vi "MainWiFi.vi"() -> ()   [LabVIEW 2018]
doc: "This example sets the RS-485 transceiver control modes for the specified port and performs a serial port read, a serial port write, or a combination of these actions. If all are selected, the VI will write the data first, read data and then close the VISA session that is opened to the port. This VI will wait until the specified number of bytes is received at the port or until a termination character is received. This example will work only with National Instruments RS-485 interfaces.\n\nThis example demonstrates the transceiver control modes available when using a National Instruments RS-485 product. When connecting one or several devices via RS-485, a user may want to cut down on the amount of wiring. Alternatively, some devices offer a certain wiring configuration that you may need to match. Determine the wiring needs of the connected serial device to determine which NI RS-485 transceiver control mode to choose.\n\nWhen you are communicating with a two-wire device, National Instruments recommends that you use the two-wire Auto Control mode. This mode handles the transmitter/receiver enabling for a two-wire connection in your hardware, so it reduces the software overhead required to perform this operation in your application program."
uses:
  estados.ctl
  mensagemFila.ctl
panel:
  in  "Port":u16=555 caption="Numeric"
  in  "IP Address":string="192.168.4.1" caption="String"
  out "elements":T1[](array[typedef])
  out "# elements in queue":i32
  out "?":T2
  in  "Power":bool
  out "SP = VP\nEscravo 2":bool
  out "SP = VP\nEscravo 1":bool
  out "Waveform Chart":T3(graph)
  in  "Sensor Escravo 2":u16(ring) caption="Ring" items=["LM35", "4 - 20 mA"]
  in  "Sensor Escravo 1":u16(ring) caption="Ring" items=["LM35", "4 - 20 mA"]
  in  "Verifica Sensor sl2":bool caption="Verifica Sensor\nEscravo 2"
  in  "Verifica Sensor sl1":bool caption="Verifica Sensor\nEscravo 1"
  in  "Envia Sensor sl2":bool caption="Seta Sensor\nEscravo 2"
  in  "Envia Sensor sl1":bool caption="Seta Sensor\nEscravo 1"
  out "Status":string caption="String"
  in  "Verifica SP sl2":bool caption="Verifica SP\nEscravo 2"
  in  "Verifica SP sl1":bool caption="Verifica SP\nEscravo 1"
  in  "SP escravo 2":u16 caption="SP Escravo 2"
  in  "Envia SP sl2":bool caption="Seta SP\nEscravo 2"
  in  "Envia SP sl1":bool caption="Seta SP\nEscravo 1"
  in  "SP escravo 1":u16 caption="SP Escravo 1"
  in  "stop":bool
  in  "dado":u16=4
  in  "opcode":u8=4 format="%.0b"
  in  "addr":u8=4 format="%.0x"
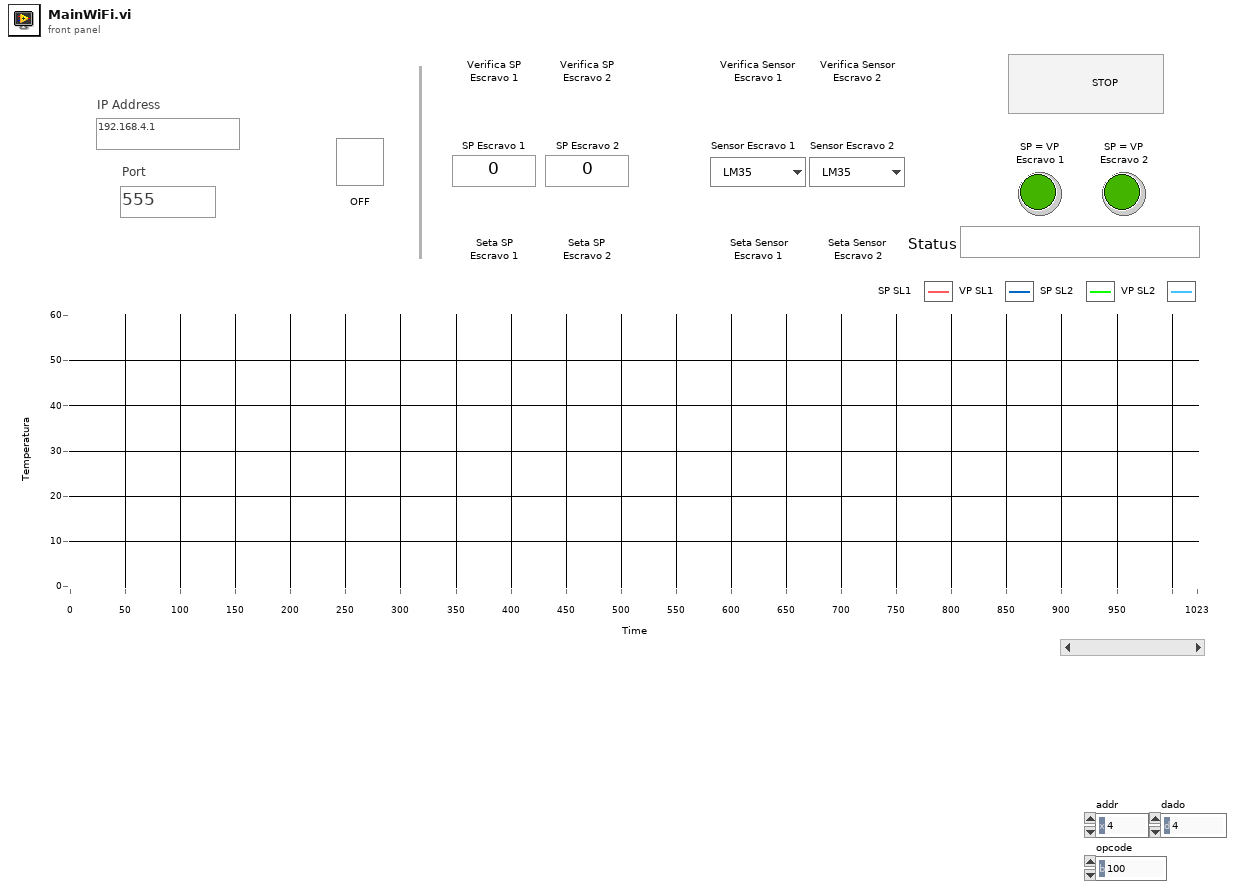
[diagram p1: front panel]
types:
  T1 = typedef "mensagemFila.ctl" = cluster{"Estado":T2, "Próximo Estado":T2, "Comando":string}
  T2 = typedef "estados.ctl" = enum16{"Idle", "Inicializa conexão", "Monta comando", "Envia comando", "Recebe resposta 1 escravo", "Recebe resposta 2 escravos", "Trata respostas", "Trata respostas 2 Escravos", "Encerra conexão", "Erro", "Stop", "Atualiza UI"}
  T3 = cluster{"plot 0":dbl, "plot 1":dbl, "plot 2":dbl, "plot 3":dbl}
  T4 = cluster{"SP escravo 1":refnum<vi>, "SP escravo 2":refnum<vi>, "Sensor Escravo 1":refnum<vi>, "Sensor Escravo 2":refnum<vi>, "SP = VP\nEscravo 1":refnum<vi>, "SP = VP\nEscravo 2":refnum<vi>, "Waveform Chart":refnum<vi>}
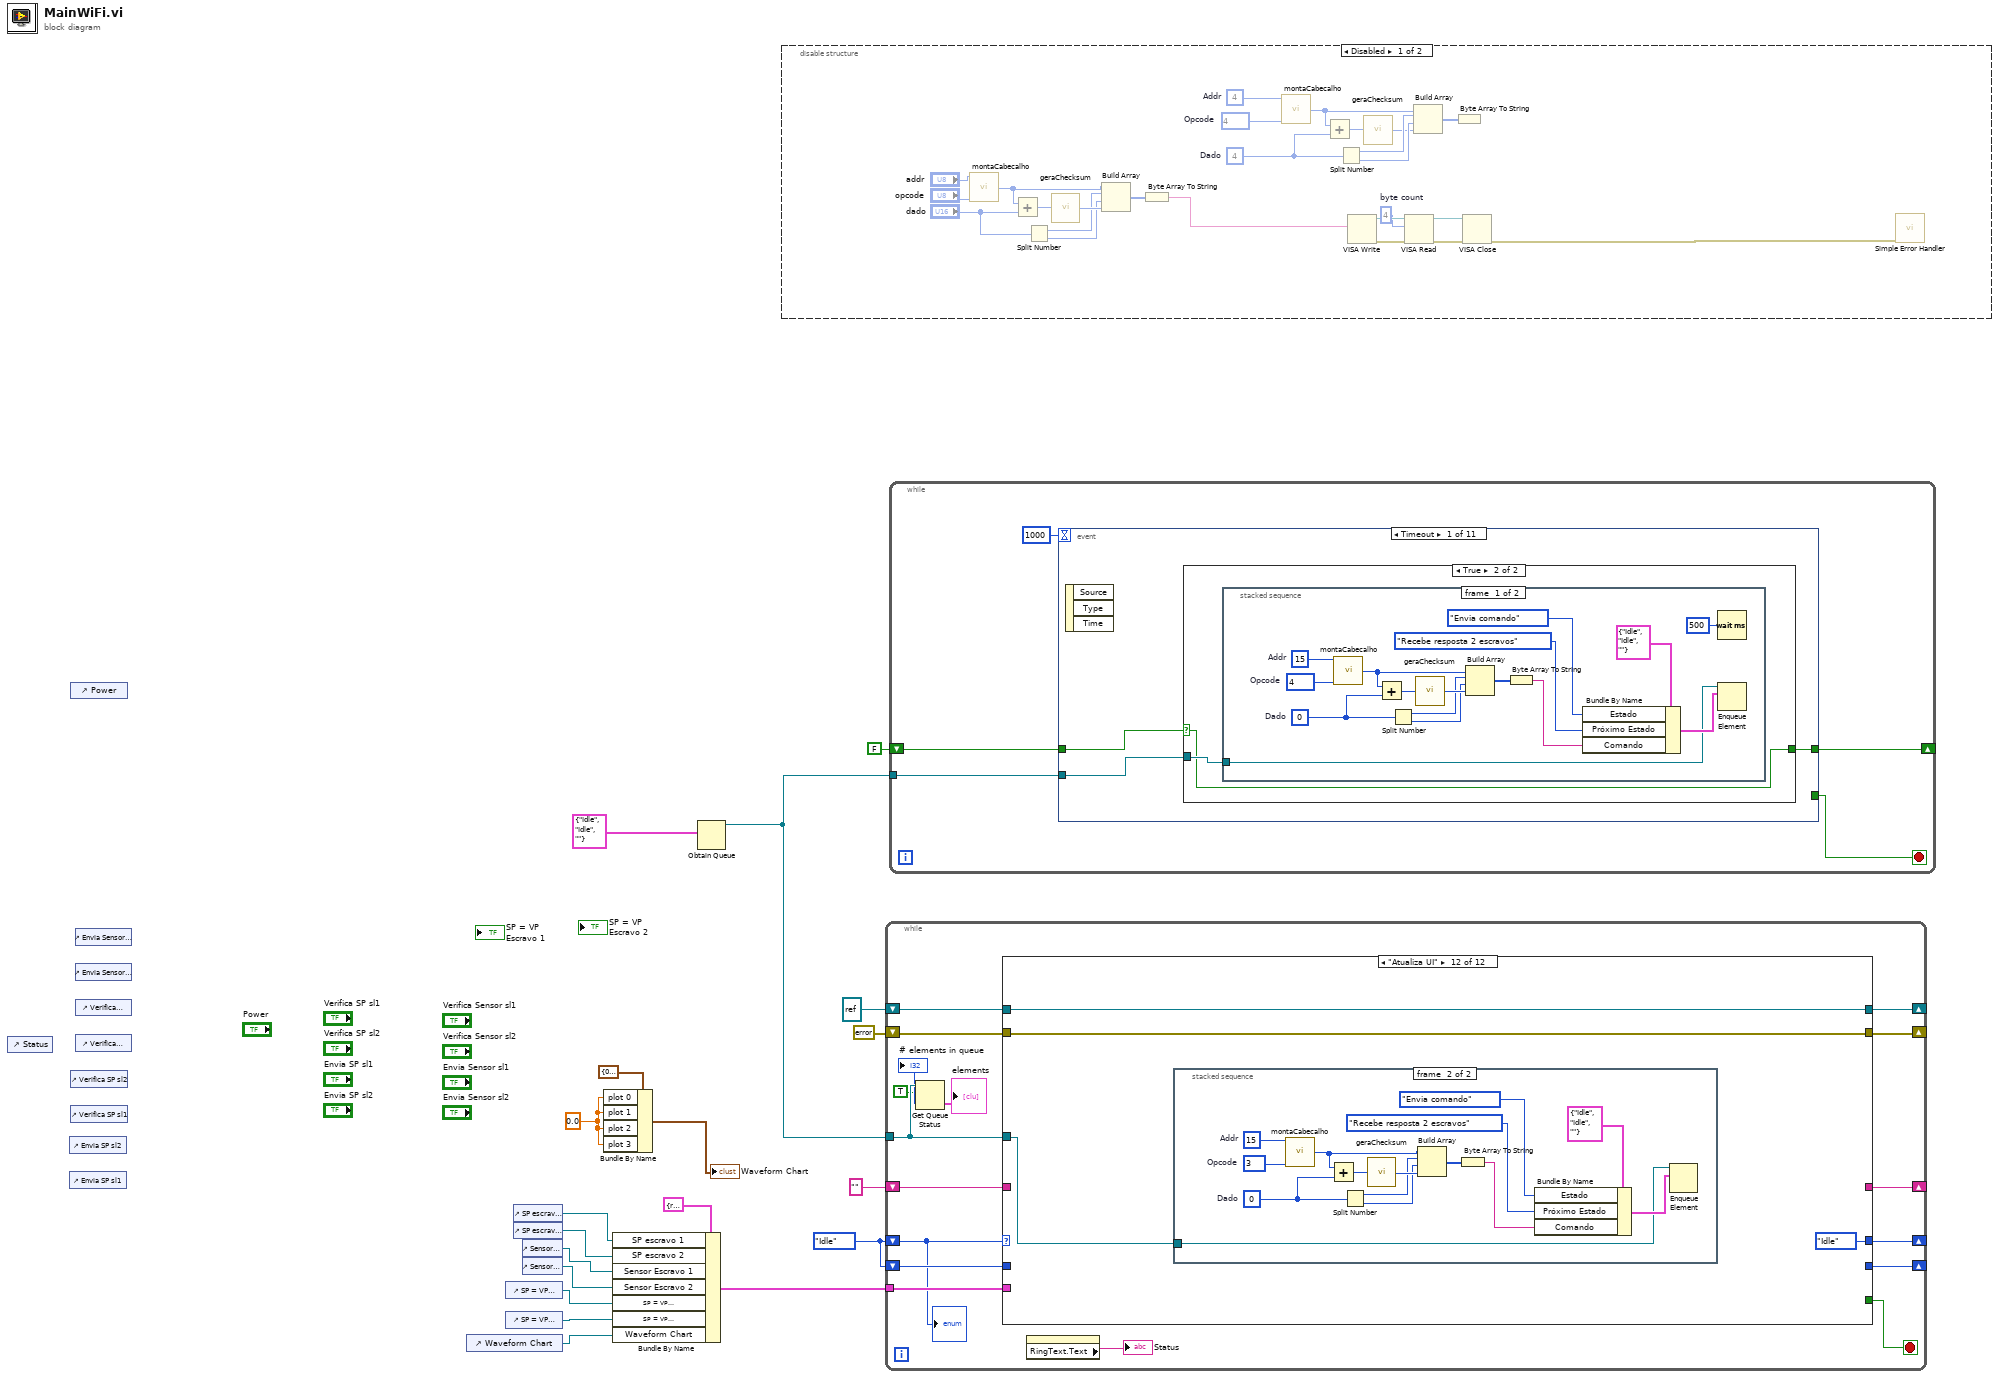
[diagram p0: block diagram]
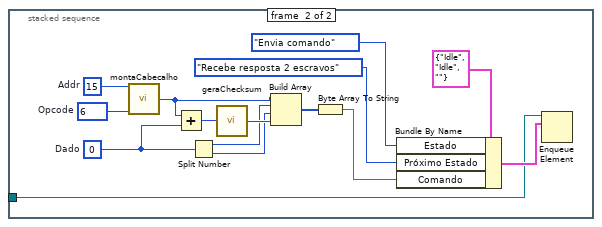
[diagram p4: hidden frame]
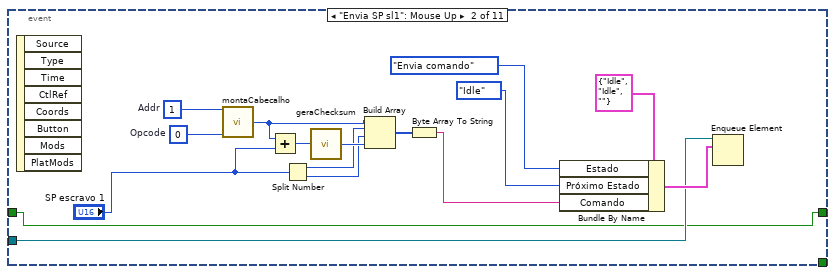
[diagram p5: hidden frame]
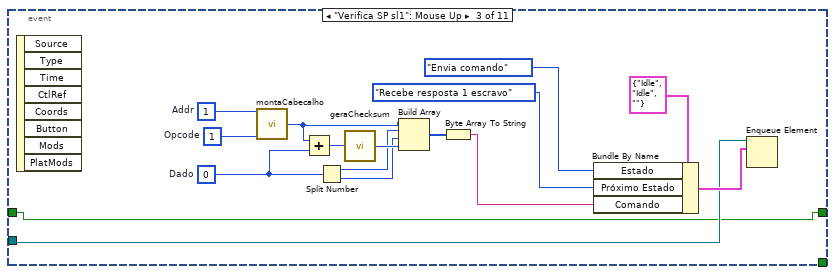
[diagram p6: hidden frame]
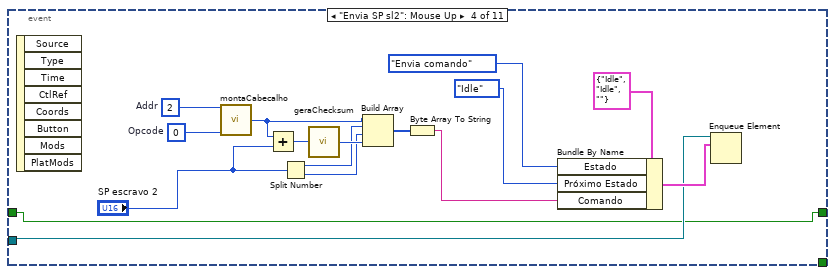
[diagram p7: hidden frame]
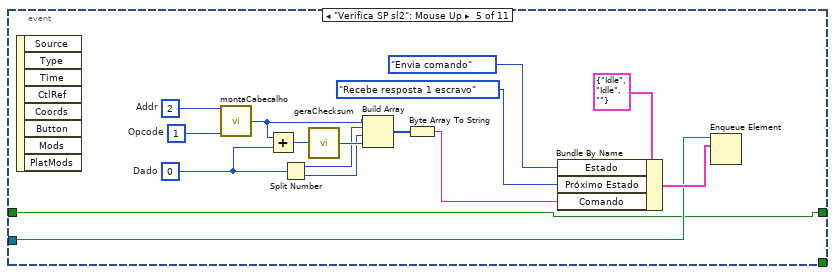
[diagram p8: hidden frame]
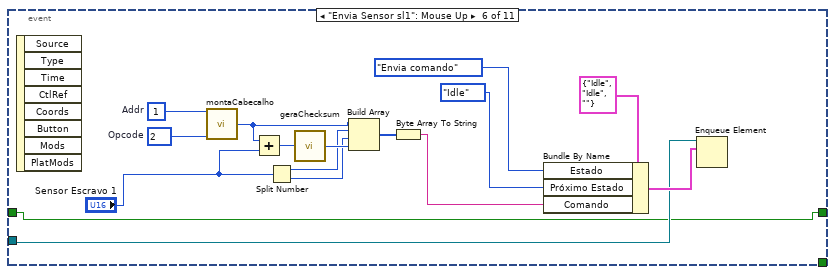
[diagram p9: hidden frame]
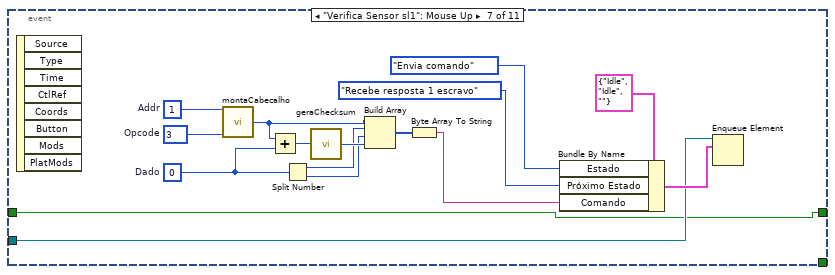
[diagram p10: hidden frame]
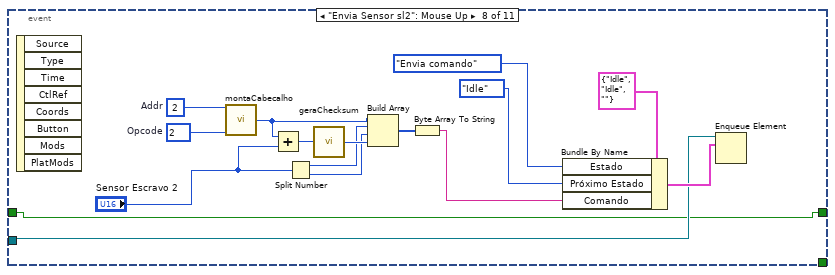
[diagram p11: hidden frame]
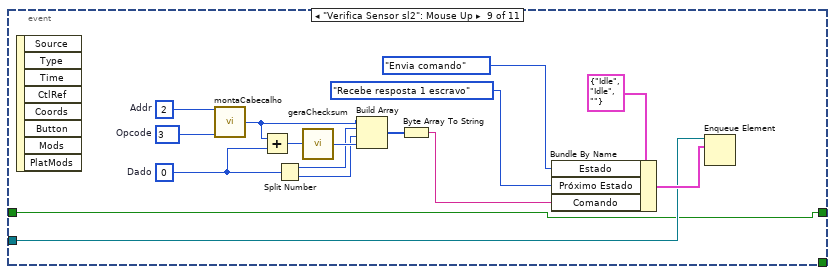
[diagram p12: hidden frame]
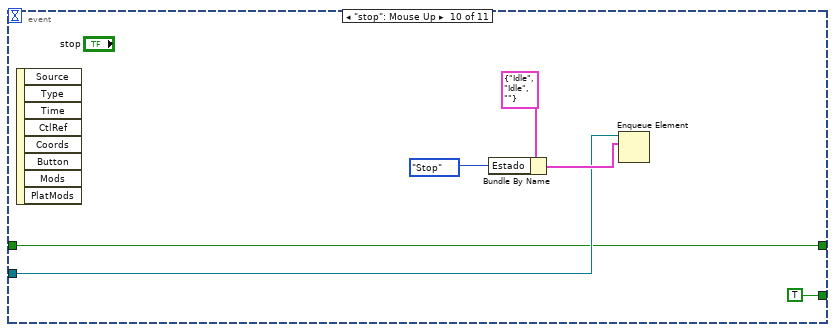
[diagram p13: hidden frame]
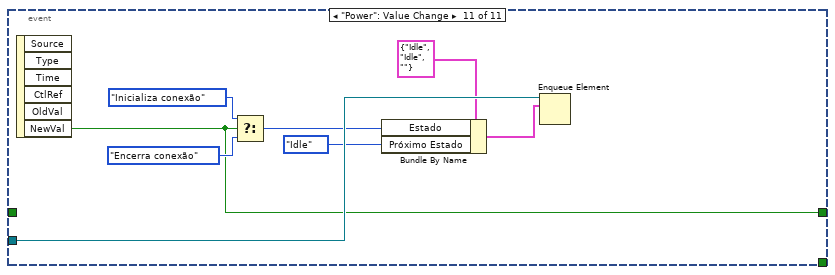
[diagram p14: hidden frame]
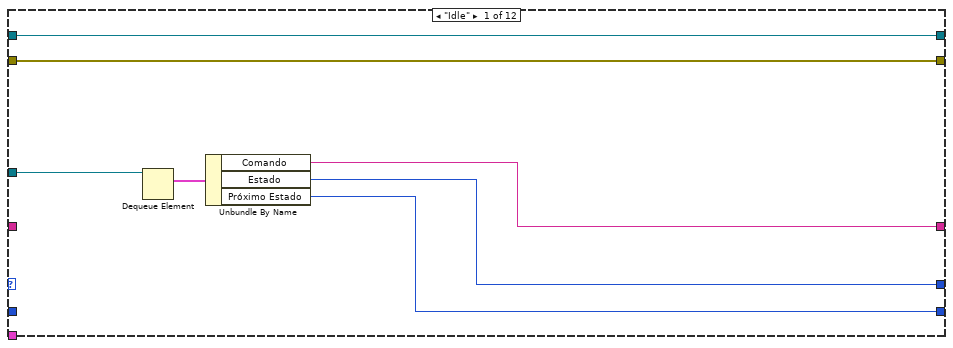
[diagram p15: hidden frame]
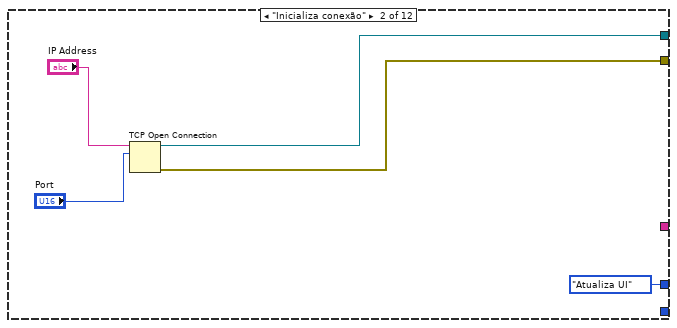
[diagram p16: hidden frame]
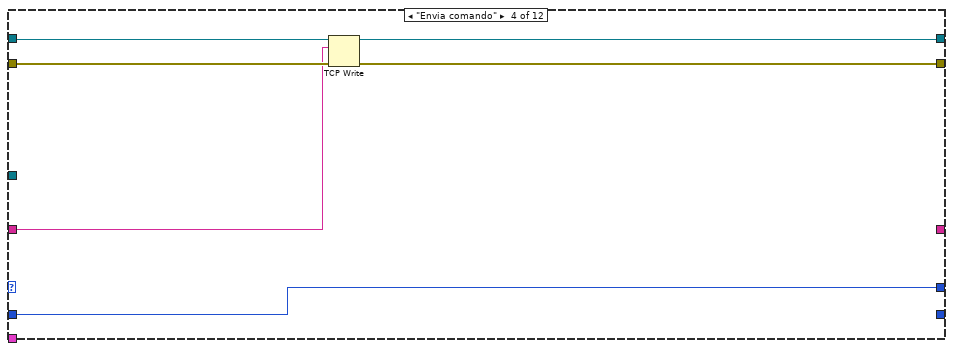
[diagram p18: hidden frame]
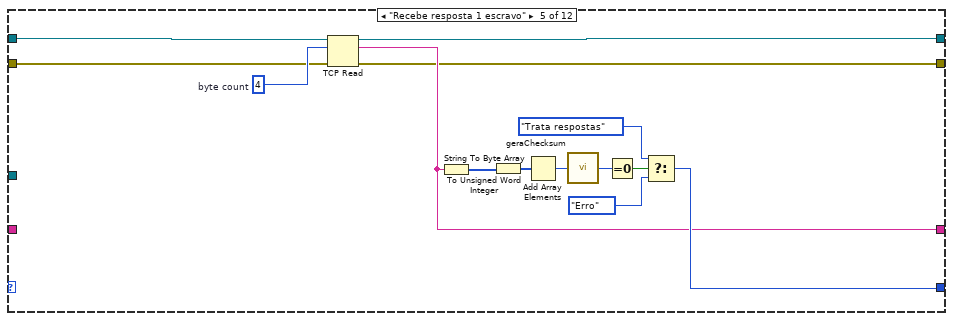
[diagram p19: hidden frame]
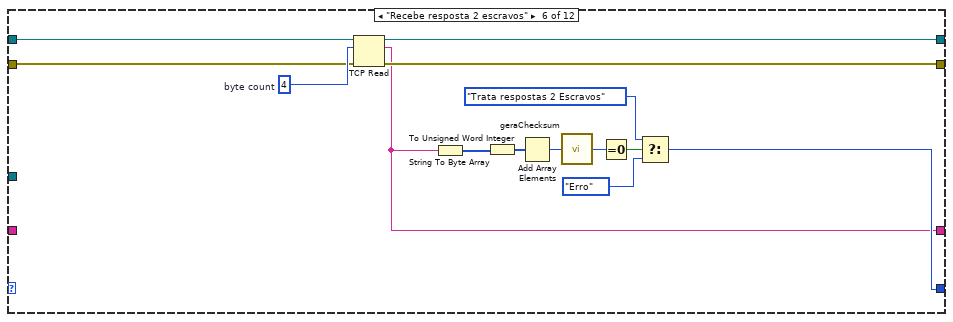
[diagram p20: hidden frame]
diagram:
  w3 = 0.0 ("element")
  w2 = estados."Idle"
  n1 = control-ref of="Status"() -> ()  [unwired: 1 out]
  n2 = control-ref of="Envia SP sl2"() -> ()  [unwired: 1 out]
  n3 = control-ref of="Envia SP sl1"() -> ()  [unwired: 1 out]
  n4 = control-ref of="Power"() -> ()  [unwired: 1 out]
  n5 = control-ref of="Verifica SP sl2"() -> ()  [unwired: 1 out]
  n6 = control-ref of="Verifica SP sl1"() -> ()  [unwired: 1 out]
  n7 = control-ref of="Envia Sensor sl2"() -> ()  [unwired: 1 out]
  n8 = control-ref of="Envia Sensor sl1"() -> ()  [unwired: 1 out]
  n9 = control-ref of="Verifica Sensor sl2"() -> ()  [unwired: 1 out]
  n10 = control-ref of="Verifica Sensor sl1"() -> ()  [unwired: 1 out]
  n11 = control-ref of="Waveform Chart"() -> (w7:refnum<vi>)
  n12 = control-ref of="SP = VP\nEscravo 1"() -> (w9:refnum<vi>)
  n13 = control-ref of="SP = VP\nEscravo 2"() -> (w8:refnum<vi>)
  n14 = control-ref of="SP escravo 1"() -> (w13:refnum<vi>)
  n15 = control-ref of="SP escravo 2"() -> (w12:refnum<vi>)
  n16 = control-ref of="Sensor Escravo 1"() -> (w11:refnum<vi>)
  n17 = control-ref of="Sensor Escravo 2"() -> (w10:refnum<vi>)
  n18 = Bundle By Name(cluster=T3 {"plot 0"=0.0, "plot 1"=0.0, "plot 2"=0.0, "plot 3"=0.0} ("input cluster"), "plot 0"=w3, "plot 1"=w3, "plot 2"=w3, "plot 3"=w3) -> (→"Waveform Chart":T3)
  n19 = Bundle By Name(cluster=T4 {"SP escravo 1"=refnum, "SP escravo 2"=refnum, "Sensor Escravo 1"=refnum, "Sensor Escravo 2"=refnum, "SP = VP\nEscravo 1"=refnum, "SP = VP\nEscravo 2"=refnum, "Waveform Chart"=refnum}, "SP escravo 1"=w13, "SP escravo 2"=w12, "Sensor Escravo 1"=w11, "Sensor Escravo 2"=w10, "SP = VP\nEscravo 1"=w9, "SP = VP\nEscravo 2"=w8, "Waveform Chart"=w7) -> (w6:T4)
  n20 = Obtain Queue(element data type=T1 {"Estado"=enum."Idle", "Próximo Estado"=enum."Idle", "Comando"=""}) -> (queue out=w17:refnum<queue>)  [unwired: 4 in, 2 out]
  n21 = disable-structure shown="Disabled" {
    frame Disabled {
      w26 = u8 4  # Addr
      w27 = u8 4  # Opcode
      w23 = u16 4  # Dado
      w39 = u32 4  # byte count
      n22 = call "montaCabecalho.vi"("addr"="addr", "opcode"="opcode") -> ("Cabeçalho"=w30:u8)  [unwired: 13 in]
      n23 = Add(x=w30, y="dado") -> (x+y=w36:u16)
      n24 = Split Number(x="dado") -> (hi(x)=w34:u8, lo(x)=w33:u8)
      n25 = call "geraChecksum.vi"("Soma"=w36) -> ("checksum"=w38:u8)  [unwired: 14 in]
      n26 = Build Array(w30, w34, w33, w38) -> (w37:u8[])
      n27 = Byte Array To String(unsigned byte array=w37) -> (string=w29:string)
      n28 = call "montaCabecalho.vi"("addr"=w26, "opcode"=w27) -> ("Cabeçalho"=w28:u8)  [unwired: 13 in]
      n29 = Add(x=w28, y=w23) -> (x+y=w22:u16)
      n30 = Split Number(x=w23) -> (hi(x)=w24:u8, lo(x)=w25:u8)
      n31 = VISA Write(write buffer=w29) -> (VISA resource name out=w44:refnum<visa-resource-name>, error out=w41:errorcluster)  [unwired: 2 in, 1 out]
      n32 = call "geraChecksum.vi"("Soma"=w22) -> ("checksum"=w20:u8)  [unwired: 14 in]
      n33 = VISA Read(VISA resource name=w44, byte count=w39, error in (no error)=w41) -> (VISA resource name out=w42:refnum<visa-resource-name>, error out=w43:errorcluster)  [unwired: 2 out]
      n34 = Build Array(w28, w24, w25, w20) -> (w21:u8[])
      n35 = Byte Array To String(unsigned byte array=w21) -> ()  [unwired: 1 out]
      n36 = VISA Close(VISA resource name=w42, error in (no error)=w43) -> (error out=w40:errorcluster)
      n37 = call <vilib>:"Simple Error Handler.vi"("error in (no error)"=w40) -> ()  [unwired: 1 in, 8 out]
    }
    frame Enabled {
    }
  }
  n38 = while {
    shift-right: [w59] -> _
    shift-left: w2 -> [w50]
    shift-right: [w58] -> _
    shift-left: errorcluster {"status"=FALSE, "code"=0, "source"=""} ("error out") -> [w60]
    shift-right: [w57] -> _
    shift-left: refnum<k5> refnum ("connection ID") -> [w61]
    shift-right: [w54] -> _
    shift-left: "" ("Dado") -> [w56]
    tunnel: w17 -> [w48]
    shift-right: [w52] -> _
    shift-left: w2 -> [w53]
    tunnel: w6 -> [w51]
    stop <- w55 stop-if-true
    n39 = Get Queue Status(queue=w48, return elements? (F)=TRUE) -> (# elements in queue=→"# elements in queue":i32, elements=→"elements":T1[])  [unwired: 1 in, 6 out]
    n40 = case shown="\"Atualiza UI\"" w50 {
      tunnel: w61 -> [w67 _ w75 w81 w85 w109 w115 w132 w136 w138 w141 w148]
      tunnel: w60 -> [w68 _ w76 w82 w95 w108 w116 w133 w137 w139 w142 w147]
      tunnel: [w63 estados."Atualiza UI" _ w77 w87 w100 estados."Idle" estados."Recebe resposta 1 escravo" _ estados."Idle" _ estados."Idle"] -> w59
      tunnel: [w68 w72 w76 w79 w83 w107 w116 w133 w135 w139 w142 w147] -> w58
      tunnel: [w67 w73 w75 w80 w84 w106 w115 w132 _ w138 w141 w148] -> w57
      tunnel: w56 -> [_ _ w74 w78 _ _ w118 w124 _ _ _ _]
      tunnel: [_ _ _ _ _ _ _ _ _ _ TRUE _] -> w55
      tunnel: w48 -> [w66 _ _ _ _ _ _ _ _ _ w143 w146]
      tunnel: [w64 _ w74 _ w86 w97 _ _ _ _ _ _] -> w54
      tunnel: w53 -> [_ _ _ w77 _ _ _ _ _ _ _ _]
      tunnel: [w62 _ _ _ _ _ _ _ _ _ _ _] -> w52
      tunnel: w51 -> [_ _ _ _ _ _ w111 w123 _ _ _ _]
      frame "Idle" {
        n41 = Dequeue Element(queue=w66) -> (element=w65:T1)  [unwired: 2 in, 3 out]
        n42 = Unbundle By Name(w65) -> ("Comando"=w64:string, "Estado"=w63:T2, "Próximo Estado"=w62:T2)
      }
      frame "Inicializa conexão" {
        n43 = TCP Open Connection(address="IP Address", remote port or service name="Port") -> (connection ID=w73:refnum<k5>, error out=w72:errorcluster)  [unwired: 3 in]
      }
      frame "Monta comando" {
      }
      frame "Envia comando" {
        n44 = TCP Write(connection ID=w81, data in=w78, error in (no error)=w82) -> (connection ID out=w80:refnum<k5>, error out=w79:errorcluster)  [unwired: 1 in, 1 out]
      }
      frame "Recebe resposta 1 escravo" {
        w96 = u32 4  # byte count
        n45 = TCP Read(connection ID=w85, bytes to read=w96, error in (no error)=w95) -> (connection ID out=w84:refnum<k5>, data out=w86:string, error out=w83:errorcluster)  [unwired: 2 in]
        n46 = String To Byte Array(string=w86) -> (unsigned byte array=w93:u8[])
        n47 = To Unsigned Word Integer(number=w93) -> (unsigned 16bit integer=w94:u16[])
        n48 = Add Array Elements(numeric array=w94) -> (sum=w92:u16)
        n49 = call "geraChecksum.vi"("Soma"=w92) -> ("checksum"=w91:u8)  [unwired: 14 in]
        n50 = Equal To 0?(x=w91) -> (x = 0?=w90:bool)
        n51 = Select(t=estados."Trata respostas", s=w90, f=estados."Erro") -> (s? t:f=w87:T2)
      }
      frame "Recebe resposta 2 escravos" {
        w110 = u32 4  # byte count
        n52 = TCP Read(connection ID=w109, bytes to read=w110, error in (no error)=w108) -> (connection ID out=w106:refnum<k5>, data out=w97:string, error out=w107:errorcluster)  [unwired: 2 in]
        n53 = String To Byte Array(string=w97) -> (unsigned byte array=w104:u8[])
        n54 = To Unsigned Word Integer(number=w104) -> (unsigned 16bit integer=w105:u16[])
        n55 = Add Array Elements(numeric array=w105) -> (sum=w103:u16)
        n56 = call "geraChecksum.vi"("Soma"=w103) -> ("checksum"=w102:u8)  [unwired: 14 in]
        n57 = Equal To 0?(x=w102) -> (x = 0?=w101:bool)
        n58 = Select(t=estados."Trata respostas 2 Escravos", s=w101, f=estados."Erro") -> (s? t:f=w100:T2)
      }
      frame "Trata respostas" {
        n59 = String To Byte Array(string=w118) -> (unsigned byte array=w122:u8[])
        n60 = Index Array(array=w122) -> (element #1=w121:u8, element #2=w120:u8, element #3=w119:u8)  [unwired: 3 in]
        n61 = call "desmontaCabecalho.vi"("cabeçalho"=w121) -> ("addr"=w112:u8, "opcode"=w113:u8)  [unwired: 13 in]
        n62 = Join Numbers(hi=w120, lo=w119) -> ((hi.lo)=w114:u16)
        n63 = call "trataMsg.vi"("addr"=w112, "opcode"=w113, "dado"=w114, "ClusterUI"=w111) -> ()  [unwired: 12 in]
      }
      frame "Trata respostas 2 Escravos" {
        n64 = String To Byte Array(string=w124) -> (unsigned byte array=w131:u8[])
        n65 = Index Array(array=w131) -> (element #1=w130:u8, element #2=w129:u8, element #3=w128:u8)  [unwired: 3 in]
        n66 = call "desmontaCabecalho.vi"("cabeçalho"=w130) -> ("addr"=w125:u8, "opcode"=w126:u8)  [unwired: 13 in]
        n67 = Join Numbers(hi=w129, lo=w128) -> ((hi.lo)=w127:u16)
        n68 = call "trataMsg.vi"("addr"=w125, "opcode"=w126, "dado"=w127, "ClusterUI"=w123) -> ()  [unwired: 12 in]
      }
      frame "Encerra conexão" {
        n69 = TCP Close Connection(connection ID=w136, error in (no error)=w137) -> (error out=w135:errorcluster)  [unwired: 1 in, 1 out]
      }
      frame "Erro" {
      }
      frame "Stop" {
        n70 = Release Queue(queue=w143) -> ()  [unwired: 2 in, 3 out]
      }
      frame "Atualiza UI" {
        n71 = stacked-sequence {
          tunnel: w146 -> [w163 w178]
          frame #0 {
            w155 = u8 15  # Addr
            w154 = u8 1  # Opcode
            w158 = u16 0  # Dado
            n72 = call "montaCabecalho.vi"("addr"=w155, "opcode"=w154) -> ("Cabeçalho"=w153:u8)  [unwired: 13 in]
            n73 = Add(x=w153, y=w158) -> (x+y=w159:u16)
            n74 = Split Number(x=w158) -> (hi(x)=w157:u8, lo(x)=w156:u8)
            n75 = call "geraChecksum.vi"("Soma"=w159) -> ("checksum"=w161:u8)  [unwired: 14 in]
            n76 = Build Array(w153, w157, w156, w161) -> (w160:u8[])
            n77 = Byte Array To String(unsigned byte array=w160) -> (string=w151:string)
            n78 = Bundle By Name(cluster=T1 {"Estado"=enum."Idle", "Próximo Estado"=enum."Idle", "Comando"=""}, "Estado"=estados."Envia comando", "Próximo Estado"=estados."Recebe resposta 2 escravos" ("Estado"), "Comando"=w151) -> (w164:T1)
            n79 = Wait (ms)(milliseconds to wait=u32 500) -> ()  [unwired: 1 out]
            n80 = Enqueue Element(queue=w163, element=w164) -> ()  [unwired: 2 in, 3 out]
          }
          frame #1 {
            w170 = u8 15  # Addr
            w169 = u8 3  # Opcode
            w173 = u16 0  # Dado
            n81 = call "montaCabecalho.vi"("addr"=w170, "opcode"=w169) -> ("Cabeçalho"=w168:u8)  [unwired: 13 in]
            n82 = Add(x=w168, y=w173) -> (x+y=w174:u16)
            n83 = Split Number(x=w173) -> (hi(x)=w172:u8, lo(x)=w171:u8)
            n84 = call "geraChecksum.vi"("Soma"=w174) -> ("checksum"=w176:u8)  [unwired: 14 in]
            n85 = Build Array(w168, w172, w171, w176) -> (w175:u8[])
            n86 = Byte Array To String(unsigned byte array=w175) -> (string=w166:string)
            n87 = Bundle By Name(cluster=T1 {"Estado"=enum."Idle", "Próximo Estado"=enum."Idle", "Comando"=""}, "Estado"=estados."Envia comando", "Próximo Estado"=estados."Recebe resposta 2 escravos" ("Estado"), "Comando"=w166) -> (w179:T1)
            n88 = Enqueue Element(queue=w178, element=w179) -> ()  [unwired: 2 in, 3 out]
          }
        }
      }
    }
    n89 = property class="Enum (strict)"() -> ("RingText.Text"=→"Status":string)  [unwired: 2 in, 2 out]
    "?" <- w50
  }
  n90 = while {
    tunnel: w17 -> [w183]
    shift-right: [w181] -> _
    shift-left: FALSE ("NewVal") -> [w180]
    stop <- w184 stop-if-true
    n91 = event shown="[0] Timeout" {
      selector: _ -> [_ _ _ _ _ _ _ _ _ _ _]
      dyn-events: _ -> [_ _ _ _ _ _ _ _ _ _ _]
      timeout: 1000 -> [_ _ _ _ _ _ _ _ _ _ _]
      tunnel: [_ _ _ _ _ _ _ _ _ TRUE _] -> w184
      tunnel: w183 -> [w187 w224 w239 w256 w271 w288 w303 w320 w335 w351 w361]
      tunnel: [w185 w222 w238 w254 w270 w286 w302 w318 w334 w350 w356] -> w181
      tunnel: w180 -> [w186 w222 w238 w254 w270 w286 w302 w318 w334 w350 _]
      event Timeout {
        n92 = event-data() -> ()  [unwired: 1 in, 3 out]
        n93 = case shown="True" w186 {
          selector: w186 -> [w188 w189]
          tunnel: w187 -> [_ w190]
          tunnel: [w188 w189] -> w185
          frame False {
          }
          frame True {
            n94 = stacked-sequence {
              tunnel: w190 -> [w205 w220]
              frame #0 {
                w197 = u8 15  # Addr
                w196 = u8 4  # Opcode
                w200 = u16 0  # Dado
                n95 = call "montaCabecalho.vi"("addr"=w197, "opcode"=w196) -> ("Cabeçalho"=w195:u8)  [unwired: 13 in]
                n96 = Add(x=w195, y=w200) -> (x+y=w201:u16)
                n97 = Split Number(x=w200) -> (hi(x)=w199:u8, lo(x)=w198:u8)
                n98 = call "geraChecksum.vi"("Soma"=w201) -> ("checksum"=w203:u8)  [unwired: 14 in]
                n99 = Build Array(w195, w199, w198, w203) -> (w202:u8[])
                n100 = Byte Array To String(unsigned byte array=w202) -> (string=w193:string)
                n101 = Bundle By Name(cluster=T1 {"Estado"=enum."Idle", "Próximo Estado"=enum."Idle", "Comando"=""}, "Estado"=estados."Envia comando", "Próximo Estado"=estados."Recebe resposta 2 escravos" ("Estado"), "Comando"=w193) -> (w206:T1)
                n102 = Wait (ms)(milliseconds to wait=u32 500) -> ()  [unwired: 1 out]
                n103 = Enqueue Element(queue=w205, element=w206) -> ()  [unwired: 2 in, 3 out]
              }
              frame #1 {
                w212 = u8 15  # Addr
                w211 = u8 6  # Opcode
                w215 = u16 0  # Dado
                n104 = call "montaCabecalho.vi"("addr"=w212, "opcode"=w211) -> ("Cabeçalho"=w210:u8)  [unwired: 13 in]
                n105 = Add(x=w210, y=w215) -> (x+y=w216:u16)
                n106 = Split Number(x=w215) -> (hi(x)=w214:u8, lo(x)=w213:u8)
                n107 = call "geraChecksum.vi"("Soma"=w216) -> ("checksum"=w218:u8)  [unwired: 14 in]
                n108 = Build Array(w210, w214, w213, w218) -> (w217:u8[])
                n109 = Byte Array To String(unsigned byte array=w217) -> (string=w208:string)
                n110 = Bundle By Name(cluster=T1 {"Estado"=enum."Idle", "Próximo Estado"=enum."Idle", "Comando"=""}, "Estado"=estados."Envia comando", "Próximo Estado"=estados."Recebe resposta 2 escravos" ("Estado"), "Comando"=w208) -> (w221:T1)
                n111 = Enqueue Element(queue=w220, element=w221) -> ()  [unwired: 2 in, 3 out]
              }
            }
          }
        }
      }
      event "Envia SP sl1": Mouse Up {
        w230 = u8 1  # Addr
        w229 = u8 0  # Opcode
        n112 = event-data() -> ()  [unwired: 1 in, 8 out]
        n113 = call "montaCabecalho.vi"("addr"=w230, "opcode"=w229) -> ("Cabeçalho"=w228:u8)  [unwired: 13 in]
        n114 = Add(x=w228, y="SP escravo 1") -> (x+y=w233:u16)
        n115 = Split Number(x="SP escravo 1") -> (hi(x)=w232:u8, lo(x)=w231:u8)
        n116 = call "geraChecksum.vi"("Soma"=w233) -> ("checksum"=w235:u8)  [unwired: 14 in]
        n117 = Build Array(w228, w232, w231, w235) -> (w234:u8[])
        n118 = Byte Array To String(unsigned byte array=w234) -> (string=w226:string)
        n119 = Bundle By Name(cluster=T1 {"Estado"=enum."Idle", "Próximo Estado"=enum."Idle", "Comando"=""}, "Estado"=estados."Envia comando", "Próximo Estado"=estados."Idle" ("Estado"), "Comando"=w226) -> (w237:T1)
        n120 = Enqueue Element(queue=w224, element=w237) -> ()  [unwired: 2 in, 3 out]
      }
      event "Verifica SP sl1": Mouse Up {
        w245 = u8 1  # Addr
        w244 = u8 1  # Opcode
        w248 = u16 0  # Dado
        n121 = event-data() -> ()  [unwired: 1 in, 8 out]
        n122 = call "montaCabecalho.vi"("addr"=w245, "opcode"=w244) -> ("Cabeçalho"=w243:u8)  [unwired: 13 in]
        n123 = Add(x=w243, y=w248) -> (x+y=w249:u16)
        n124 = Split Number(x=w248) -> (hi(x)=w247:u8, lo(x)=w246:u8)
        n125 = call "geraChecksum.vi"("Soma"=w249) -> ("checksum"=w251:u8)  [unwired: 14 in]
        n126 = Build Array(w243, w247, w246, w251) -> (w250:u8[])
        n127 = Byte Array To String(unsigned byte array=w250) -> (string=w241:string)
        n128 = Bundle By Name(cluster=T1 {"Estado"=enum."Idle", "Próximo Estado"=enum."Idle", "Comando"=""}, "Estado"=estados."Envia comando", "Próximo Estado"=estados."Recebe resposta 1 escravo" ("Estado"), "Comando"=w241) -> (w253:T1)
        n129 = Enqueue Element(queue=w239, element=w253) -> ()  [unwired: 2 in, 3 out]
      }
      event "Envia SP sl2": Mouse Up {
        w262 = u8 2  # Addr
        w261 = u8 0  # Opcode
        n130 = event-data() -> ()  [unwired: 1 in, 8 out]
        n131 = call "montaCabecalho.vi"("addr"=w262, "opcode"=w261) -> ("Cabeçalho"=w260:u8)  [unwired: 13 in]
        n132 = Add(x=w260, y="SP escravo 2") -> (x+y=w265:u16)
        n133 = Split Number(x="SP escravo 2") -> (hi(x)=w264:u8, lo(x)=w263:u8)
        n134 = call "geraChecksum.vi"("Soma"=w265) -> ("checksum"=w267:u8)  [unwired: 14 in]
        n135 = Build Array(w260, w264, w263, w267) -> (w266:u8[])
        n136 = Byte Array To String(unsigned byte array=w266) -> (string=w258:string)
        n137 = Bundle By Name(cluster=T1 {"Estado"=enum."Idle", "Próximo Estado"=enum."Idle", "Comando"=""}, "Estado"=estados."Envia comando", "Próximo Estado"=estados."Idle" ("Estado"), "Comando"=w258) -> (w269:T1)
        n138 = Enqueue Element(queue=w256, element=w269) -> ()  [unwired: 2 in, 3 out]
      }
      event "Verifica SP sl2": Mouse Up {
        w277 = u8 2  # Addr
        w276 = u8 1  # Opcode
        w280 = u16 0  # Dado
        n139 = event-data() -> ()  [unwired: 1 in, 8 out]
        n140 = call "montaCabecalho.vi"("addr"=w277, "opcode"=w276) -> ("Cabeçalho"=w275:u8)  [unwired: 13 in]
        n141 = Add(x=w275, y=w280) -> (x+y=w281:u16)
        n142 = Split Number(x=w280) -> (hi(x)=w279:u8, lo(x)=w278:u8)
        n143 = call "geraChecksum.vi"("Soma"=w281) -> ("checksum"=w283:u8)  [unwired: 14 in]
        n144 = Build Array(w275, w279, w278, w283) -> (w282:u8[])
        n145 = Byte Array To String(unsigned byte array=w282) -> (string=w273:string)
        n146 = Bundle By Name(cluster=T1 {"Estado"=enum."Idle", "Próximo Estado"=enum."Idle", "Comando"=""}, "Estado"=estados."Envia comando", "Próximo Estado"=estados."Recebe resposta 1 escravo" ("Estado"), "Comando"=w273) -> (w285:T1)
        n147 = Enqueue Element(queue=w271, element=w285) -> ()  [unwired: 2 in, 3 out]
      }
      event "Envia Sensor sl1": Mouse Up {
        w294 = u8 1  # Addr
        w293 = u8 2  # Opcode
        n148 = event-data() -> ()  [unwired: 1 in, 8 out]
        n149 = call "montaCabecalho.vi"("addr"=w294, "opcode"=w293) -> ("Cabeçalho"=w292:u8)  [unwired: 13 in]
        n150 = Add(x=w292, y="Sensor Escravo 1") -> (x+y=w297:u16)
        n151 = Split Number(x="Sensor Escravo 1") -> (hi(x)=w296:u8, lo(x)=w295:u8)
        n152 = call "geraChecksum.vi"("Soma"=w297) -> ("checksum"=w299:u8)  [unwired: 14 in]
        n153 = Build Array(w292, w296, w295, w299) -> (w298:u8[])
        n154 = Byte Array To String(unsigned byte array=w298) -> (string=w290:string)
        n155 = Bundle By Name(cluster=T1 {"Estado"=enum."Idle", "Próximo Estado"=enum."Idle", "Comando"=""}, "Estado"=estados."Envia comando", "Próximo Estado"=estados."Idle" ("Estado"), "Comando"=w290) -> (w301:T1)
        n156 = Enqueue Element(queue=w288, element=w301) -> ()  [unwired: 2 in, 3 out]
      }
      event "Verifica Sensor sl1": Mouse Up {
        w309 = u8 1  # Addr
        w308 = u8 3  # Opcode
        w312 = u16 0  # Dado
        n157 = event-data() -> ()  [unwired: 1 in, 8 out]
        n158 = call "montaCabecalho.vi"("addr"=w309, "opcode"=w308) -> ("Cabeçalho"=w307:u8)  [unwired: 13 in]
        n159 = Add(x=w307, y=w312) -> (x+y=w313:u16)
        n160 = Split Number(x=w312) -> (hi(x)=w311:u8, lo(x)=w310:u8)
        n161 = call "geraChecksum.vi"("Soma"=w313) -> ("checksum"=w315:u8)  [unwired: 14 in]
        n162 = Build Array(w307, w311, w310, w315) -> (w314:u8[])
        n163 = Byte Array To String(unsigned byte array=w314) -> (string=w305:string)
        n164 = Bundle By Name(cluster=T1 {"Estado"=enum."Idle", "Próximo Estado"=enum."Idle", "Comando"=""}, "Estado"=estados."Envia comando", "Próximo Estado"=estados."Recebe resposta 1 escravo" ("Estado"), "Comando"=w305) -> (w317:T1)
        n165 = Enqueue Element(queue=w303, element=w317) -> ()  [unwired: 2 in, 3 out]
      }
      event "Envia Sensor sl2": Mouse Up {
        w326 = u8 2  # Addr
        w325 = u8 2  # Opcode
        n166 = event-data() -> ()  [unwired: 1 in, 8 out]
        n167 = call "montaCabecalho.vi"("addr"=w326, "opcode"=w325) -> ("Cabeçalho"=w324:u8)  [unwired: 13 in]
        n168 = Add(x=w324, y="Sensor Escravo 2") -> (x+y=w329:u16)
        n169 = Split Number(x="Sensor Escravo 2") -> (hi(x)=w328:u8, lo(x)=w327:u8)
        n170 = call "geraChecksum.vi"("Soma"=w329) -> ("checksum"=w331:u8)  [unwired: 14 in]
        n171 = Build Array(w324, w328, w327, w331) -> (w330:u8[])
        n172 = Byte Array To String(unsigned byte array=w330) -> (string=w322:string)
        n173 = Bundle By Name(cluster=T1 {"Estado"=enum."Idle", "Próximo Estado"=enum."Idle", "Comando"=""}, "Estado"=estados."Envia comando", "Próximo Estado"=estados."Idle" ("Estado"), "Comando"=w322) -> (w333:T1)
        n174 = Enqueue Element(queue=w320, element=w333) -> ()  [unwired: 2 in, 3 out]
      }
      event "Verifica Sensor sl2": Mouse Up {
        w341 = u8 2  # Addr
        w340 = u8 3  # Opcode
        w339 = u16 0  # Dado
        n175 = event-data() -> ()  [unwired: 1 in, 8 out]
        n176 = call "montaCabecalho.vi"("addr"=w341, "opcode"=w340) -> ("Cabeçalho"=w343:u8)  [unwired: 13 in]
        n177 = Add(x=w343, y=w339) -> (x+y=w346:u16)
        n178 = Split Number(x=w339) -> (hi(x)=w345:u8, lo(x)=w344:u8)
        n179 = call "geraChecksum.vi"("Soma"=w346) -> ("checksum"=w348:u8)  [unwired: 14 in]
        n180 = Build Array(w343, w345, w344, w348) -> (w347:u8[])
        n181 = Byte Array To String(unsigned byte array=w347) -> (string=w342:string)
        n182 = Bundle By Name(cluster=T1 {"Estado"=enum."Idle", "Próximo Estado"=enum."Idle", "Comando"=""}, "Estado"=estados."Envia comando", "Próximo Estado"=estados."Recebe resposta 1 escravo" ("Estado"), "Comando"=w342) -> (w349:T1)
        n183 = Enqueue Element(queue=w335, element=w349) -> ()  [unwired: 2 in, 3 out]
      }
      event "stop": Mouse Up {
        n184 = event-data() -> ()  [unwired: 1 in, 8 out]
        n185 = Bundle By Name(cluster=T1 {"Estado"=enum."Idle", "Próximo Estado"=enum."Idle", "Comando"=""}, "Estado"=estados."Stop") -> (w354:T1)
        n186 = Enqueue Element(queue=w351, element=w354) -> ()  [unwired: 2 in, 3 out]
      }
      event "Power": Value Change {
        n187 = event-data() -> ("NewVal"=w356:bool)  [unwired: 1 in, 5 out]
        n188 = Select(t=estados."Inicializa conexão", s=w356, f=estados."Encerra conexão") -> (s? t:f=w360:T2)
        n189 = Bundle By Name(cluster=T1 {"Estado"=enum."Idle", "Próximo Estado"=enum."Idle", "Comando"=""}, "Estado"=w360, "Próximo Estado"=estados."Idle") -> (w358:T1)
        n190 = Enqueue Element(queue=w361, element=w358) -> ()  [unwired: 2 in, 3 out]
      }
    }
  }
